vi "IR LearnEvent Example.vi"() -> ()   [LabVIEW 2012, in "Phidget IR.lvlib"]
uses:
  <instrlib>/Phidgets/Phidget IR/Phidget IR.lvlib
  <instrlib>/Phidgets/Phidget IR/Public/CodeInfo.ctl
  <instrlib>/Phidgets/Phidget IR/Public/IRStart.vi
  <instrlib>/Phidgets/Phidget IR/Public/IRClose.vi
  <instrlib>/Phidgets/Phidget Common/Phidget Common.lvlib
panel:
  out "codeInfo out":T1={"bitCount"=0, "encoding"=1, "length"=1, "gap"=0, "trail"=0, "header[0]"=0, "header[1]"=0, "one[0]"=0, "one[1]"=0, "zero[0]"=0, "zero[1]"=0, "repeat[0]"=0, "repeat[1]"=0, "repeat[2]"=0, "repeat[3]"=0, "repeat[4]"=0, "repeat[5]"=0, "repeat[6]"=0, "repeat[7]"=0, "repeat[8]"=0, "repeat[9]"=0, "repeat[10]"=0, "repeat[11]"=0, "repeat[12]"=0, "repeat[13]"=0, "repeat[14]"=0, "repeat[15]"=0, "repeat[16]"=0, "repeat[17]"=0, "repeat[18]"=0, "repeat[19]"=0, "repeat[20]"=0, "repeat[21]"=0, "repeat[22]"=0, "repeat[23]"=0, "repeat[24]"=0, "repeat[25]"=0, "minRepeat"=0, "dutyCycle"=0.0, "carrierFrequency"=0, "toggleMask[0]"=0, "toggleMask[1]"=0, "toggleMask[2]"=0, "toggleMask[3]"=0, "toggleMask[4]"=0, "toggleMask[5]"=0, "toggleMask[6]"=0, "toggleMask[7]"=0, "toggleMask[8]"=0, "toggleMask[9]"=0, "toggleMask[10]"=0, "toggleMask[11]"=0, "toggleMask[12]"=0, "toggleMask[13]"=0, "toggleMask[14]"=0, "toggleMask[15]"=0, "toggleMask[16]"=0, "toggleMask[17]"=0, "toggleMask[18]"=0, "toggleMask[19]"=0, "toggleMask[20]"=0, "toggleMask[21]"=0, "toggleMask[22]"=0, "toggleMask[23]"=0, "toggleMask[24]"=0, "toggleMask[25]"=0, "toggleMask[26]"=0, "toggleMask[27]"=0, "toggleMask[28]"=0, "toggleMask[29]"=0, "toggleMask[30]"=0, "toggleMask[31]"=0, "toggleMask[32]"=0} {"encoding" items=["IR_ENCODING_UNKNOWN"=1, "IR_ENCODING_SPACE"=2, "IR_ENCODING_PULSE"=3, "IR_ENCODING_BIPHASE"=4, "IR_ENCODING_RC5"=5, "IR_ENCODING_RC6"=6]; "length" items=["IR_LENGTH_UNKNOWN"=1, "IR_LENGTH_CONSTANT"=2, "IR_LENGTH_VARIABLE"=3]}
  out "Code String":string
  in  "stop":bool
  out "Serial Number Return":i32
  in  "Device Info":T2={"Serial Number"=-1, "Channel"=0, "Port"=0}
  out "error out":errorcluster
  # "Be sure to use this stop button to stop the program.\nIf you use the \"Abort Execution\" button, you will\nneed to use PhidgetResetLibrary.vi or restart Labview \nin order for any Phidgets to work."
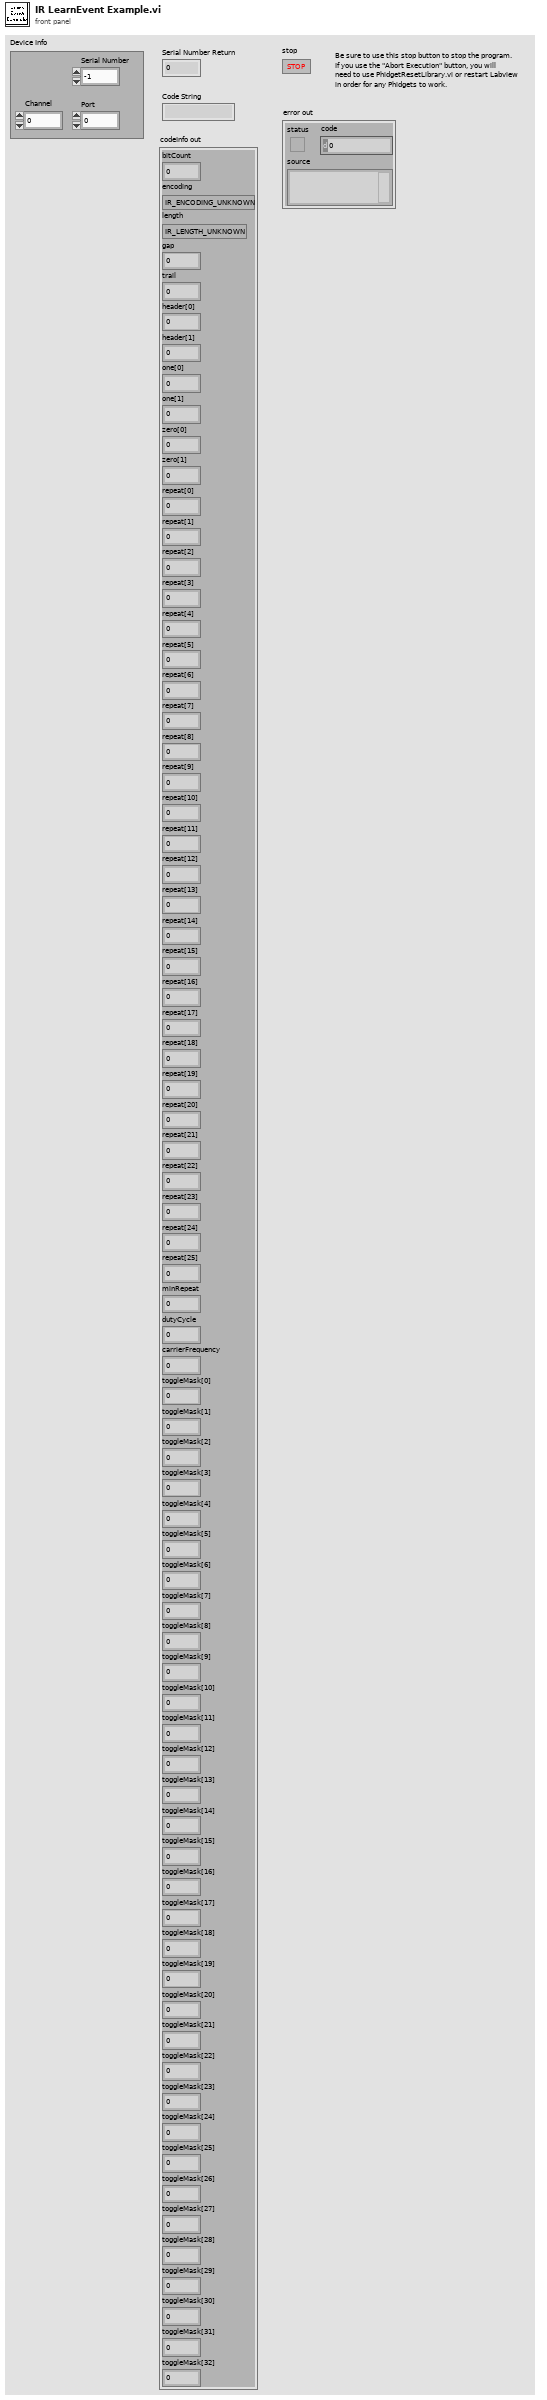
[diagram p1: front panel]
types:
  T1 = typedef "Phidget IR.lvlib/CodeInfo.ctl" = cluster{"bitCount":u32, "encoding":u32, "length":u32, "gap":u32, "trail":u32, "header[0]":u32, "header[1]":u32, "one[0]":u32, "one[1]":u32, "zero[0]":u32, "zero[1]":u32, "repeat[0]":u32, "repeat[1]":u32, "repeat[2]":u32, "repeat[3]":u32, "repeat[4]":u32, "repeat[5]":u32, "repeat[6]":u32, "repeat[7]":u32, "repeat[8]":u32, "repeat[9]":u32, "repeat[10]":u32, "repeat[11]":u32, "repeat[12]":u32, "repeat[13]":u32, "repeat[14]":u32, "repeat[15]":u32, "repeat[16]":u32, "repeat[17]":u32, "repeat[18]":u32, "repeat[19]":u32, "repeat[20]":u32, "repeat[21]":u32, "repeat[22]":u32, "repeat[23]":u32, "repeat[24]":u32, "repeat[25]":u32, "minRepeat":u32, "dutyCycle":dbl, "carrierFrequency":u32, "toggleMask[0]":i8, "toggleMask[1]":i8, "toggleMask[2]":i8, "toggleMask[3]":i8, "toggleMask[4]":i8, "toggleMask[5]":i8, "toggleMask[6]":i8, "toggleMask[7]":i8, "toggleMask[8]":i8, "toggleMask[9]":i8, "toggleMask[10]":i8, "toggleMask[11]":i8, "toggleMask[12]":i8, "toggleMask[13]":i8, "toggleMask[14]":i8, "toggleMask[15]":i8, "toggleMask[16]":i8, "toggleMask[17]":i8, "toggleMask[18]":i8, "toggleMask[19]":i8, "toggleMask[20]":i8, "toggleMask[21]":i8, "toggleMask[22]":i8, "toggleMask[23]":i8, "toggleMask[24]":i8, "toggleMask[25]":i8, "toggleMask[26]":i8, "toggleMask[27]":i8, "toggleMask[28]":i8, "toggleMask[29]":i8, "toggleMask[30]":i8, "toggleMask[31]":i8, "toggleMask[32]":i8}
  T2 = cluster{"Serial Number":i32, "Channel":i32, "Port":i32}
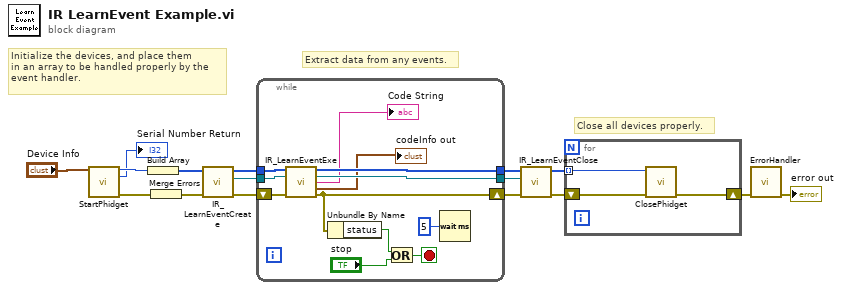
[diagram p0: block diagram]
diagram:
  # "Close all devices properly."
  # "Extract data from any events."
  # "Initialize the devices, and place them\nin an array to be handled properly by the\nevent handler."
  n1 = call-poly <instrlib>:"StartPhidget.vi"("Device Info"="Device Info") -> ("Phidget ID"=w5:u64, "Serial Number Return"=→"Serial Number Return":i32, "error out"=w1:errorcluster)  [unwired: 11 in, 1 out]
  n2 = Build Array(w5) -> (w16:u64[])
  n3 = Merge Errors(w1) -> (w7:errorcluster)
  n4 = call <instrlib>:"IR_LearnEventCreate.vi"("error in (no error)"=w7, "Devices In"=w16) -> ("error out"=w9:errorcluster, "Event Registration Refnum"=w14:refnum<event-registration>, "Devices Out"=w15:u64[])  [unwired: 7 in]
  n5 = while {
    tunnel: w15 -> [w28]
    tunnel: w14 -> [w23]
    tunnel: [w27] -> w11
    shift-right: [w22] -> w10
    shift-left: w9 -> [w26]
    tunnel: [w24] -> w3
    stop <- w21 stop-if-true
    n6 = call <instrlib>:"IR_LearnEventExe.vi"("Devices In"=w28, "Event Registration Refnum In"=w23, "error in (no error)"=w26) -> ("Devices Out"=w24:u64[], "Event Registration Refnum Out"=w27:refnum<event-registration>, "Code String"=→"Code String":string, "codeInfo"=→"codeInfo out":T1, "error out"=w22:errorcluster)  [unwired: 5 in, 3 out]
    n7 = Unbundle By Name(w22) -> ("status"=w19:bool)
    n8 = Or(x=w19, y="stop") -> (x .or. y?=w21:bool)
    n9 = Wait (ms)(milliseconds to wait=u32 5) -> ()  [unwired: 1 out]
  }
  n10 = call <instrlib>:"IR_LearnEventClose.vi"("error in (no error)"=w10, "Event Registration Refnum In"=w11, "Devices In"=w3) -> ("error out"=w6:errorcluster, "Devices Out"=w4:u64[])  [unwired: 7 in]
  n11 = for {
    tunnel: w4 -> [w29] mode=indexing
    shift-right: [w31] -> w13
    shift-left: w6 -> [w30]
    n12 = call-poly <instrlib>:"ClosePhidget.vi"("error in"=w30, "Device In"=w29) -> ("error out"=w31:errorcluster)  [unwired: 9 in]
  }
  n13 = call <instrlib>:"ErrorHandler.vi"("error in"=w13) -> ("error out"=→"error out":errorcluster)  [unwired: 9 in, 1 out]
